vi "open.vi"() -> (0 "error out":errorcluster, 3 "connection data":variant)   [LabVIEW 2011]
uses:
  remaining_string.vi
panel:
  in  "cancel connect":bool
  out "error out 2":errorcluster
  # "Connecting to target ...."
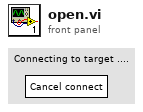
[diagram p1: front panel]
types:
  T1 = enum16{"Channel 1", "Channel 2", "Channel 3", "Real-Time Agent"}
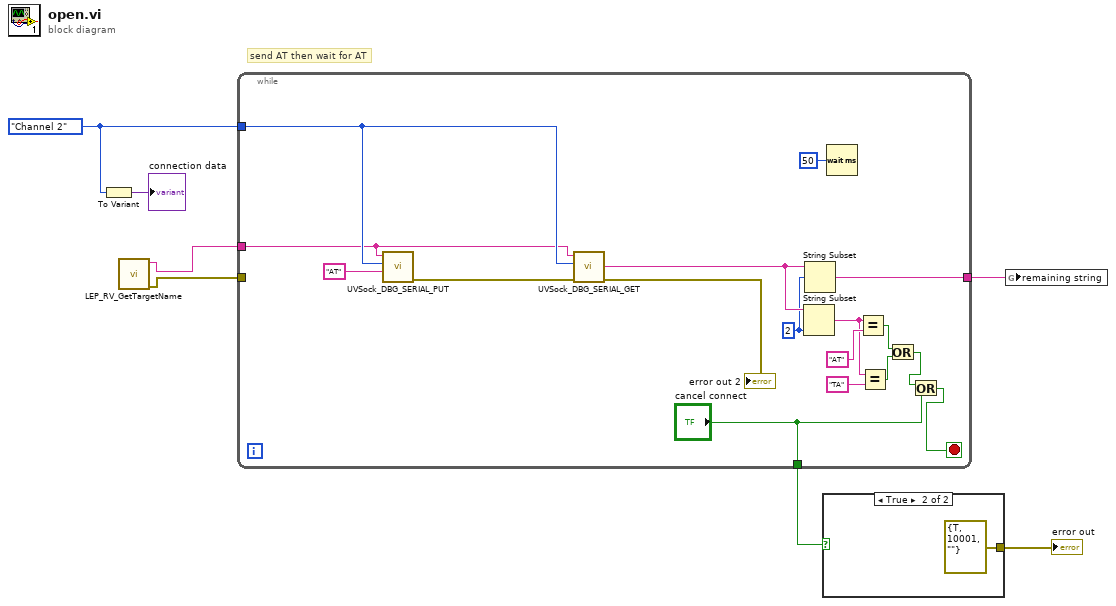
[diagram p0: block diagram]
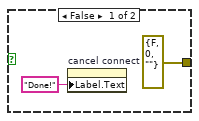
[diagram p2: hidden frame]
diagram:
  w4 = T1."Channel 2" ("Channel")
  # "send AT then wait for AT"
  n1 = To Variant(anything=w4) -> (Variant=→"connection data":variant)
  n2 = call "LEP_RV_GetTargetName.vi"() -> ("error out"=w1:errorcluster, "Target Name"=w2:string)  [unwired: 10 in]
  n3 = while {
    tunnel: ["cancel connect"] -> w5
    tunnel: w4 -> [w9]
    tunnel: [w12] -> w3
    tunnel: w1 -> [_]
    tunnel: w2 -> [w8]
    stop <- w17 stop-if-true
    w13 = 2 ("length (rest)")
    n4 = call "UVSock_DBG_SERIAL_PUT.vi"("Serial Data"="AT", "Channel"=w9, "Target"=w8) -> ("error out"=w16:errorcluster)  [unwired: 8 in]
    n5 = call "UVSock_DBG_SERIAL_GET.vi"("error in (no error)"=w16, "Channel"=w9, "Target"=w8) -> ("error out"=→"error out 2":errorcluster, "Serial Data"=w14:string)  [unwired: 6 in, 1 out]
    n6 = String Subset(string=w14, length (rest)=w13) -> (substring=w22:string)  [unwired: 1 in]
    n7 = String Subset(string=w14, offset (0)=w13) -> (substring=w12:string)  [unwired: 1 in]
    n8 = Wait (ms)(milliseconds to wait=u32 50) -> ()  [unwired: 1 out]
    n9 = Equal?(x=w22, y="AT") -> (x = y?=w20:bool)
    n10 = Equal?(x=w22, y="TA") -> (x = y?=w19:bool)
    n11 = Or(x=w20, y=w19) -> (x .or. y?=w18:bool)
    n12 = Or(x=w18, y="cancel connect") -> (x .or. y?=w17:bool)
  }
  n13 = case shown="True" w5 {
    tunnel: [errorcluster {"status"=FALSE, "code"=0, "source"=""} ("error out") errorcluster {"status"=TRUE, "code"=10001, "source"=""} ("error out")] -> w6
    frame False {
      n14 = property on="cancel connect" class="Bool"("Label.Text"="Done!") -> ()  [unwired: 2 in, 2 out]
    }
    frame True {
    }
  }
  "error out" <- w6
  n15 = global write "remaining_string.vi" "remaining string"(w3) -> ()
